vi "Pusher_Client_SendData.vi"(8 "ErrIn":errorcluster, 10 "data":string, 11 "Client in":refnum<class "Client.lvclass">) -> (0 "ErrOut":errorcluster, 3 "Client out":refnum<class "Client.lvclass">)   [LabVIEW 2009, in "Client.lvclass"]
uses:
  Client.lvclass
  Client.lvclass/Client.ctl
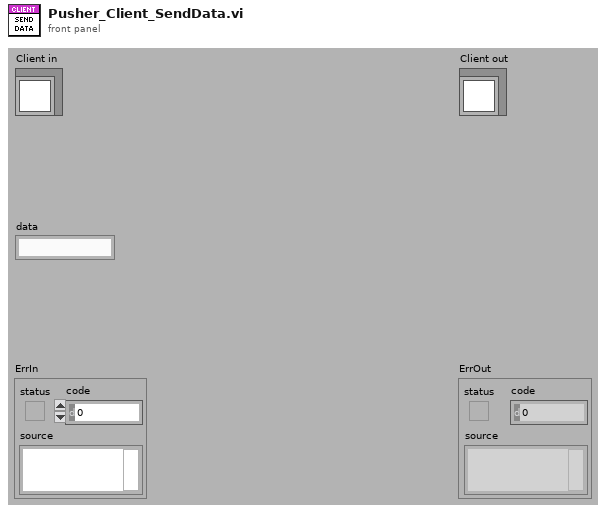
[diagram p1: front panel]
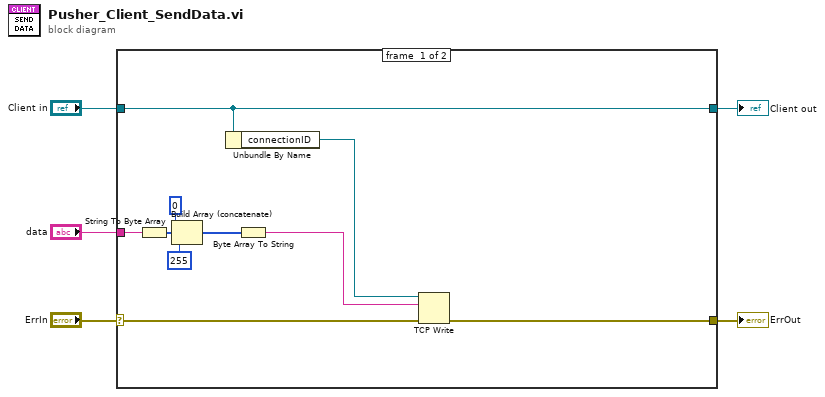
[diagram p0: block diagram]
diagram:
  n1 = case shown="No Error" "ErrIn" {
    selector: "ErrIn" -> [w10 w17]
    tunnel: [w6 w17] -> w4
    tunnel: [w9 w16] -> w2
    tunnel: "Client in" -> [w9 w16]
    tunnel: "data" -> [w11 _]
    frame #0 {
      n2 = String To Byte Array(string=w11) -> (unsigned byte array=w13:u8[])
      n3 = Build Array (concatenate)(u8 0, w13, u8 255) -> (w12:u8[])
      n4 = Unbundle By Name(w9) -> ("connectionID"=w8:refnum<k5>)
      n5 = Byte Array To String(unsigned byte array=w12) -> (string=w7:string)
      n6 = TCP Write(connection ID=w8, data in=w7, error in (no error)=w10) -> (error out=w6:errorcluster)  [unwired: 1 in, 2 out]
    }
    frame #1 {
    }
  }
  "ErrOut" <- w4
  "Client out" <- w2
